vi "Destroy.vi"(0 "reference in":refnum<class "ArrayIterator.lvclass">, 5 "error in (no error)":errorcluster) -> (14 "reference out":refnum<class "ArrayIterator.lvclass">, 19 "error out":errorcluster)   [LabVIEW 2015, in "ArrayIterator.lvclass"]
uses:
  ArrayIterator.lvclass
  Association/iRobotDebugSystem/Browers/Iterator/Interface Iterator/Iterator.lvclass
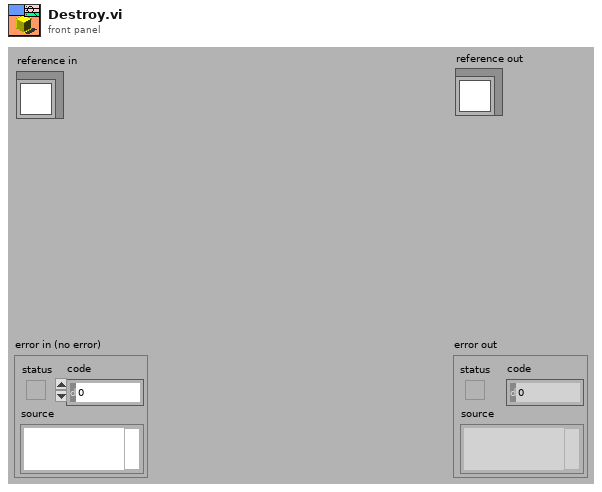
[diagram p1: front panel]
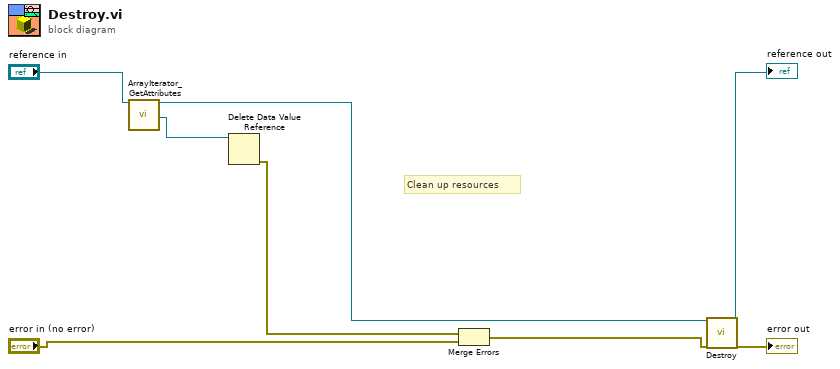
[diagram p0: block diagram]
diagram:
  # "Clean up resources"
  n1 = call "ArrayIterator_GetAttributes.vi"("reference in"="reference in") -> ("reference out"=w2:refnum<class "ArrayIterator.lvclass">, "DataRef"=w5:refnum<data-value>)  [unwired: 15 in, 2 out]
  n2 = Delete Data Value Reference(data value reference=w5) -> (error out=w3:errorcluster)  [unwired: 1 in, 1 out]
  n3 = Merge Errors(w3, "error in (no error)") -> (w1:errorcluster)
  n4 = call-parent "Destroy.vi"("reference in"=w2, "error in (no error)"=w1) -> ("reference out"=→"reference out":refnum<class "ArrayIterator.lvclass">, "error out"=→"error out":errorcluster)  [unwired: 16 in]
